vi "Get measurementservice_ACIRData.vi"(8 "error in (no error)":errorcluster, 11 "gRPCid":T4) -> (0 "error out":errorcluster, 2 "Message Data":T1, 3 "gRPCid out":T4)   [LabVIEW 2019, in "OCV3.lvlib" / "OCV3.lvclass"]
uses:
  OCV3.lvclass
  gRPC lvSupport/Server API/typeDefs/grpcId.ctl
  measurementservice_ACIRData_Data.ctl
  measurementservice_ACIRRaw/measurementservice_ACIRRaw_Data.ctl
  measurementservice_ErrorOut/measurementservice_ErrorOut_Data.ctl
  a51dd2a7-b5c1-4c09-9df4-8cd9d3bd0c19.vi
  gRPC lvSupport/Server API/Server/Get Server DLL Path.vi
  gRPC lvSupport/gprc-lvsupport.lvlib
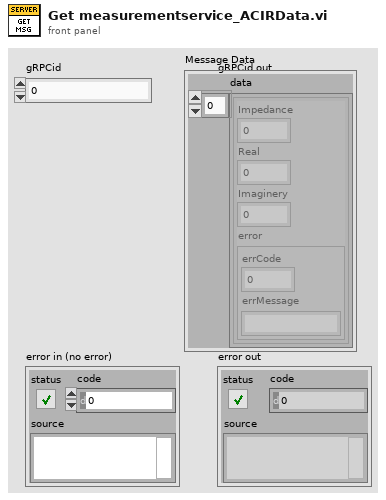
[diagram p1: front panel]
types:
  T1 = typedef "OCV3.lvlib/OCV3.lvclass/measurementservice_ACIRData_Data.ctl" = cluster{"data":T2[]}
  T2 = typedef "OCV3.lvlib/OCV3.lvclass/measurementservice_ACIRRaw_Data.ctl" = cluster{"Impedance":sgl, "Real":sgl, "Imaginery":sgl, "error":T3}
  T3 = typedef "OCV3.lvlib/OCV3.lvclass/measurementservice_ErrorOut_Data.ctl" = cluster{"errCode":i32, "errMessage":string}
  T4 = typedef "OCV3.lvlib/gprc-lvsupport.lvlib/grpcId.ctl" = u64
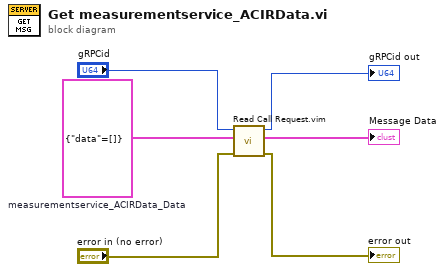
[diagram p0: block diagram]
diagram:
  w2 = T1 {"data"=[]}  # measurementservice_ACIRData_Data
  n1 = call "Read Call Request.vim"("error in (no error)"="error in (no error)", "Data Type"=w2, "gRPCid in"="gRPCid") -> ("error out"=→"error out":errorcluster, "Request Data"=→"Message Data":T1, "gRPCid out"=→"gRPCid out":T4)  [unwired: 6 in]
